vi "rename seq channel writer or reader.vi"(6 "new action channel":refnum<class "TBM channel.lvclass">, 7 "owner ID":string, 8 "error in":errorcluster, 9 "old action channel":refnum<class "TBM channel.lvclass">, 10 "seq channel":refnum<class "TBM channel.lvclass">, 11 "engine configuration in":refnum<class "base TBM sequencer configuration.lvclass">) -> (0 "error out":errorcluster, 3 "engine configuration out":refnum<class "base TBM sequencer configuration.lvclass">)   [LabVIEW 2014, in "base TBM sequencer configuration.lvclass"]
uses:
  base TBM sequencer configuration.lvclass
  <vilib>/NI/Tag Bus Module Framework/channel/TBM channel.lvclass
  <vilib>/NI/Tag Bus/tag/tag descriptor.lvclass/tag descriptor.ctl
  base TBM sequencer configuration.lvclass/base TBM sequencer configuration.ctl
  <vilib>/NI/Tag Bus Module Framework/channel/TBM channel.lvclass/TBM channel.ctl
  <vilib>/NI/Tag Bus/tag/read tag name.vi
  <vilib>/NI/Tag Bus Module Framework/channel/Read channel classification.vi
  <vilib>/NI/Configuration Framework/NISE_CEF_TreeControl.lvlib
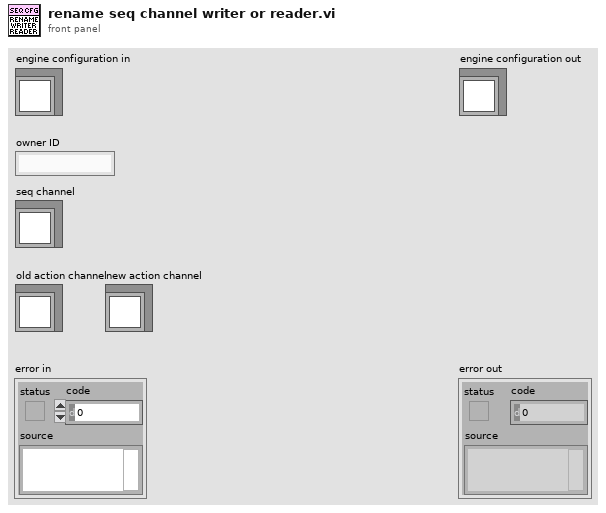
[diagram p1: front panel]
types:
  T1 = typedef "base TBM sequencer configuration.lvclass/Tag Info.ctl" = cluster{"Channel":refnum<class "TBM channel.lvclass">, "Writers":string[], "Readers":string[], "Owning ID":string}
  T2 = typedef "TBM channel.lvclass/channel classification.ctl" = enum16{"input data", "output data", "processing parameter", "processing result"}
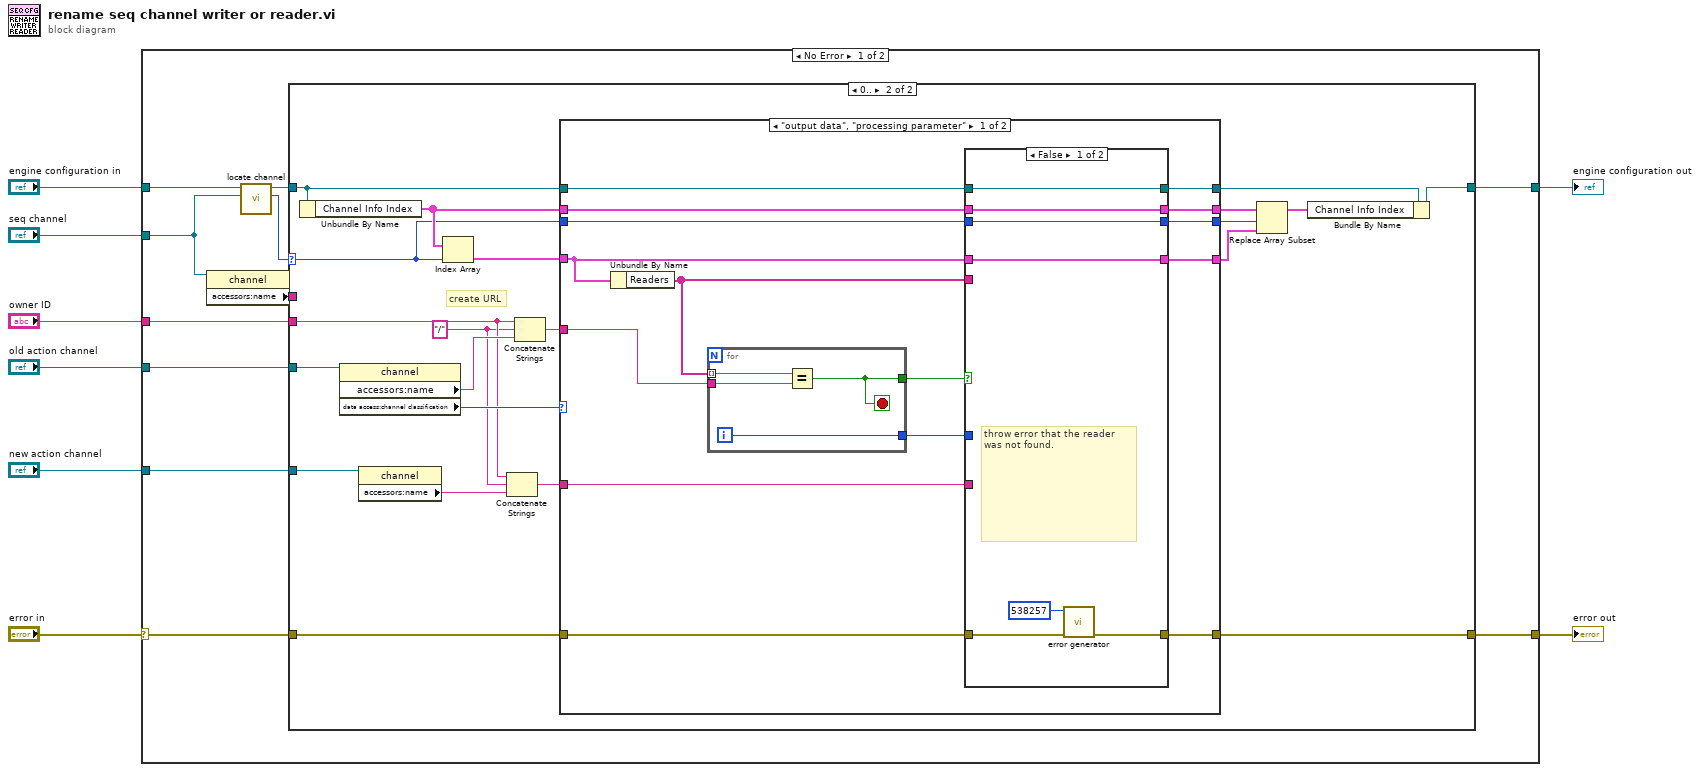
[diagram p0: block diagram]
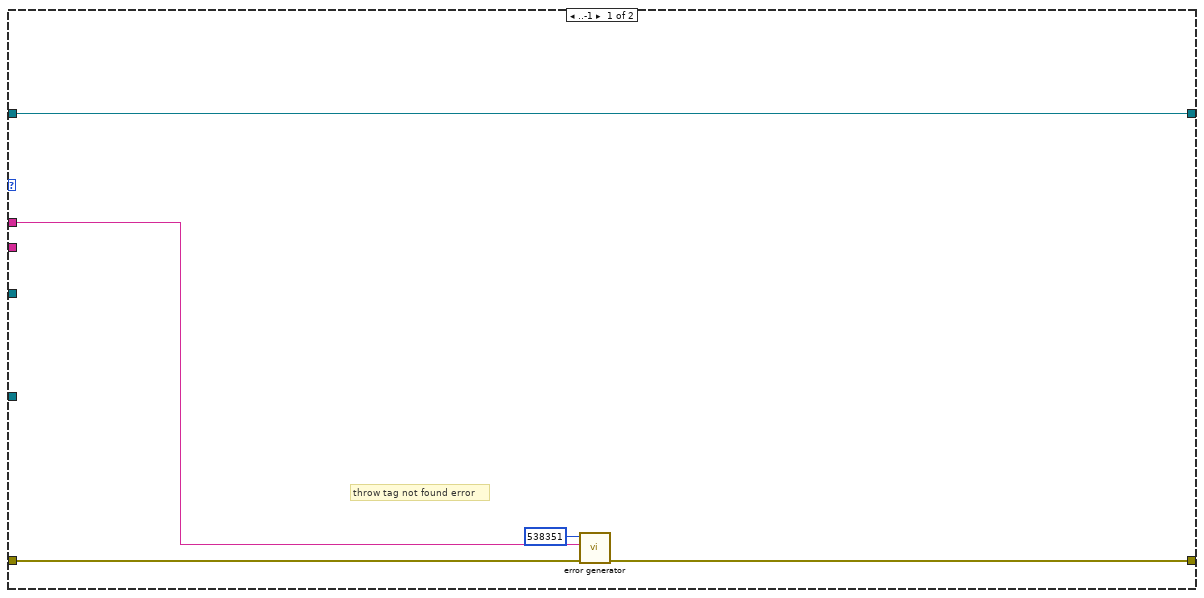
[diagram p2: hidden frame]
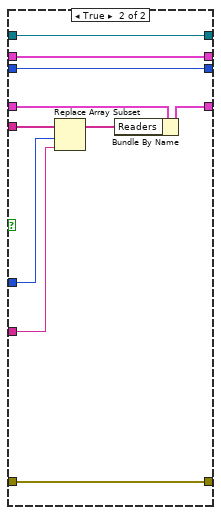
[diagram p3: hidden frame]
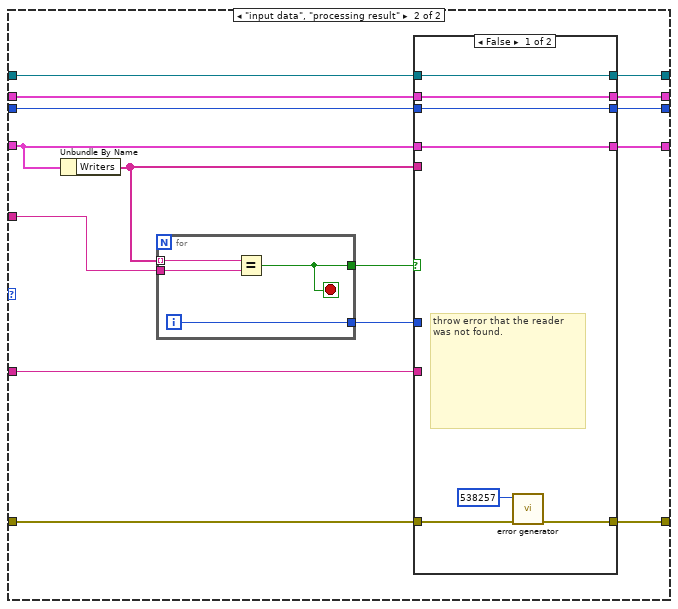
[diagram p4: hidden frame]
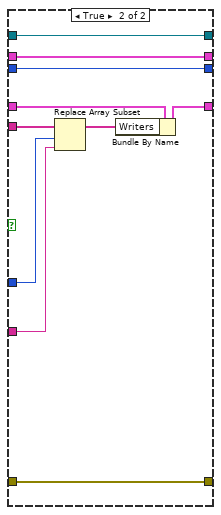
[diagram p5: hidden frame]
diagram:
  n1 = case shown="No Error" "error in" {
    selector: "error in" -> [w15 w119]
    tunnel: [w13 w119] -> w7
    tunnel: [w12 w118] -> w5
    tunnel: "engine configuration in" -> [w19 w118]
    tunnel: "seq channel" -> [w10 _]
    tunnel: "owner ID" -> [w16 _]
    tunnel: "old action channel" -> [w17 _]
    tunnel: "new action channel" -> [w11 _]
    frame No Error {
      n2 = property class="channel"(reference=w10) -> ("accessors:name"=w9:string)  [unwired: 1 in, 2 out]
      n3 = call "locate channel.vi"("tag descriptor"=w10, "sequencer config in"=w19) -> ("index"=w14:i32, "sequencer config out"=w18:refnum<class "base TBM sequencer configuration.lvclass">)  [unwired: 8 in]
      n4 = case shown="0.." w14 {
        selector: w14 -> [_ w38]
        tunnel: w18 -> [w24 w37]
        tunnel: w17 -> [_ w45]
        tunnel: w16 -> [_ w28]
        tunnel: w15 -> [w22 w40]
        tunnel: [w21 w36] -> w13
        tunnel: [w24 w30] -> w12
        tunnel: w11 -> [_ w29]
        tunnel: w9 -> [w20 _]
        frame ..-1 {
          # "throw tag not found error"
          n5 = call <vilib>:"error generator.vi"("error in"=w22, "append error message"=w20, "error code (0)"=538351) -> ("error out"=w21:errorcluster)  [unwired: 6 in]
        }
        frame 0.. {
          w27 = "/" ("string")
          # "create URL"
          n6 = Unbundle By Name(w37) -> ("Channel Info Index"=w39:T1[])
          n7 = property class="channel"(reference=w45) -> ("accessors:name"=w44:string, "data access:channel classification"=w43:T2)  [unwired: 1 in, 2 out]
          n8 = property class="channel"(reference=w29) -> ("accessors:name"=w26:string)  [unwired: 1 in, 2 out]
          n9 = Index Array(array=w39, index=w38) -> (element=w41:T1)
          n10 = Concatenate Strings(w28, w27, w26) -> (w25:string)
          n11 = Concatenate Strings(w28, w27, w44) -> (w42:string)
          n12 = case shown="\"output data\", \"processing parameter\"" w43 {
            tunnel: w42 -> [w58 w94]
            tunnel: w41 -> [w57 w93]
            tunnel: w40 -> [w53 w89]
            tunnel: w39 -> [w50 w86]
            tunnel: w38 -> [w48 w84]
            tunnel: w37 -> [w56 w92]
            tunnel: [w55 w91] -> w32
            tunnel: [w54 w90] -> w33
            tunnel: [w52 w88] -> w36
            tunnel: [w51 w87] -> w34
            tunnel: [w49 w85] -> w35
            tunnel: w25 -> [w46 w82]
            frame "output data", "processing parameter" {
              n13 = Unbundle By Name(w57) -> ("Readers"=w59:string[])
              n14 = for {
                tunnel: w59 -> [w80] mode=indexing
                tunnel: w58 -> [w81]
                tunnel: [w79] -> w60
                tunnel: [w78] -> w47
                i -> [w78]
                stop <- w79 stop-if-true
                n15 = Equal?(x=w80, y=w81) -> (x = y?=w79:bool)
              }
              n16 = case shown="False" w60 {
                tunnel: w59 -> [_ w71]
                tunnel: w57 -> [w66 w77]
                tunnel: w56 -> [w67 w76]
                tunnel: [w67 w76] -> w55
                tunnel: [w66 w75] -> w54
                tunnel: w53 -> [w62 w74]
                tunnel: [w61 w74] -> w52
                tunnel: [w65 w73] -> w51
                tunnel: w50 -> [w65 w73]
                tunnel: [w64 w72] -> w49
                tunnel: w48 -> [w64 w72]
                tunnel: w47 -> [_ w69]
                tunnel: w46 -> [_ w68]
                frame False {
                  # "throw error that the reader was not found."
                  n17 = call <vilib>:"error generator.vi"("error in"=w62, "error code (0)"=538257) -> ("error out"=w61:errorcluster)  [unwired: 7 in]
                }
                frame True {
                  n18 = Replace Array Subset(array=w71, new element=w68, index=w69) -> (w70:string[])
                  n19 = Bundle By Name(cluster=w77, "Readers"=w70) -> (w75:T1)
                }
              }
            }
            frame "input data", "processing result" {
              n20 = Unbundle By Name(w93) -> ("Writers"=w95:string[])
              n21 = for {
                tunnel: w95 -> [w116] mode=indexing
                tunnel: w94 -> [w117]
                tunnel: [w115] -> w96
                tunnel: [w114] -> w83
                i -> [w114]
                stop <- w115 stop-if-true
                n22 = Equal?(x=w116, y=w117) -> (x = y?=w115:bool)
              }
              n23 = case shown="False" w96 {
                tunnel: w95 -> [_ w107]
                tunnel: w93 -> [w102 w113]
                tunnel: w92 -> [w103 w112]
                tunnel: [w103 w112] -> w91
                tunnel: [w102 w111] -> w90
                tunnel: w89 -> [w98 w110]
                tunnel: [w97 w110] -> w88
                tunnel: [w101 w109] -> w87
                tunnel: w86 -> [w101 w109]
                tunnel: [w100 w108] -> w85
                tunnel: w84 -> [w100 w108]
                tunnel: w83 -> [_ w105]
                tunnel: w82 -> [_ w104]
                frame False {
                  # "throw error that the reader was not found."
                  n24 = call <vilib>:"error generator.vi"("error in"=w98, "error code (0)"=538257) -> ("error out"=w97:errorcluster)  [unwired: 7 in]
                }
                frame True {
                  n25 = Replace Array Subset(array=w107, new element=w104, index=w105) -> (w106:string[])
                  n26 = Bundle By Name(cluster=w113, "Writers"=w106) -> (w111:T1)
                }
              }
            }
          }
          n27 = Replace Array Subset(array=w34, new element=w33, index=w35) -> (w31:T1[])
          n28 = Bundle By Name(cluster=w32, "Channel Info Index"=w31) -> (w30:refnum<class "base TBM sequencer configuration.lvclass">)
        }
      }
    }
    frame Error {
    }
  }
  "error out" <- w7
  "engine configuration out" <- w5
